vi "json Member Names - string path.vi"(8 "error in (no error)":errorcluster, 10 "path":string, 11 "JSON Document in":refnum<class "JSON Document.lvclass">) -> (0 "error out":errorcluster, 2 "Member Names":string[](array[string]), 3 "JSON Document out":refnum<class "JSON Document.lvclass">)   [LabVIEW 2015, in "JSON Document.lvclass"]
uses:
  JSON Document.lvclass
  JSON Document.lvclass/JSON Document.ctl
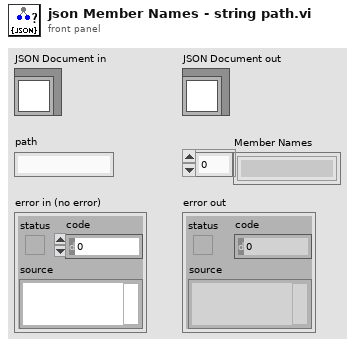
[diagram p1: front panel]
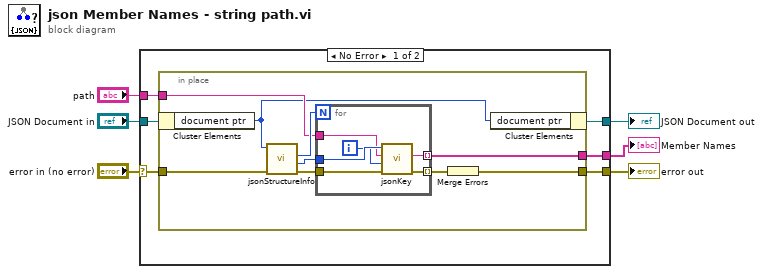
[diagram p0: block diagram]
diagram:
  n1 = case shown="No Error" "error in (no error)" {
    selector: "error in (no error)" -> [w10 w29]
    tunnel: [w7 w29] -> w5
    tunnel: [w9 w28] -> w3
    tunnel: "JSON Document in" -> [w12 w28]
    tunnel: "path" -> [w11 _]
    tunnel: [w8 _] -> w1
    frame No Error {
      n2 = in-place {
        in-place-border: w11 -> [w18]
        in-place-border: w10 -> [w21]
        in-place-border: [w17] -> w8
        in-place-border: [w13] -> w7
        n3 = in-place-cluster #1(w12) -> ("document ptr"=w16:i64)
        n4 = call "jsonStructureInfo.vi"("error in (no error)"=w21, "d in"=w16) -> ("error out"=w15:errorcluster, "value out"=w19:i64, "count"=w20:i32)  [unwired: 6 in, 1 out]
        n5 = for {
          N: w20 -> [_]
          tunnel: w19 -> [w27]
          tunnel: w18 -> [w25]
          tunnel: [w24] -> w17 mode=indexing
          tunnel: w15 -> [w23]
          tunnel: [w22] -> w14 mode=indexing
          i -> [w26]
          n6 = call "jsonKey.vi"("error in (no error)"=w23, "index"=w26, "path"=w25, "d in"=w27) -> ("error out"=w22:errorcluster, "key"=w24:string)  [unwired: 5 in, 1 out]
        }
        n7 = Merge Errors(w14) -> (w13:errorcluster)
        n8 = in-place-cluster #1("document ptr"=w16) -> (w9:refnum<class "JSON Document.lvclass">)
      }
    }
    frame Error {
    }
  }
  "error out" <- w5
  "JSON Document out" <- w3
  "Member Names" <- w1
